vi "To CSV File.vi"(8 "error in (no error)":errorcluster, 9 "Path":path, 10 "engine configuration":refnum<class "engine configuration.lvclass">, 11 "DAQmx Module Editor Node in":refnum<class "DAQmx Module Editor Node.lvclass">) -> (0 "error out":errorcluster, 3 "DAQmx Module Editor Node out":refnum<class "DAQmx Module Editor Node.lvclass">)   [LabVIEW 2014, in "DAQmx Module Editor Node.lvclass"]
uses:
  DAQmx Module Editor Node.lvclass
  <vilib>/NI/Module Execution Interface/Engine Configuration/engine configuration.lvclass
  module/configuration/DAQmx Module Configuration.lvclass
  <vilib>/NI/Configuration Framework/serializable configuration/NISE_CEF_serializable configuration.lvclass/NISE_CEF_serializable configuration.ctl
  module/configuration/DAQmx Module Configuration.lvclass/DAQmx Module Configuration.ctl
  <vilib>/NI/Tag Bus/tag/tag descriptor.lvclass/tag descriptor.ctl
  <vilib>/Utility/LVClass/Get LV Class Name.vi
  <vilib>/NI/Configuration Framework/error generator/NISE_error generator.vi
  <vilib>/NI/Configuration Framework/serializable configuration/NISE_CEF_serializable configuration.lvclass
  <vilib>/NI/Tag Bus Module Framework/channel/TBM channel.lvclass
  <vilib>/NI/Tag Bus/tag/tag descriptor.lvclass
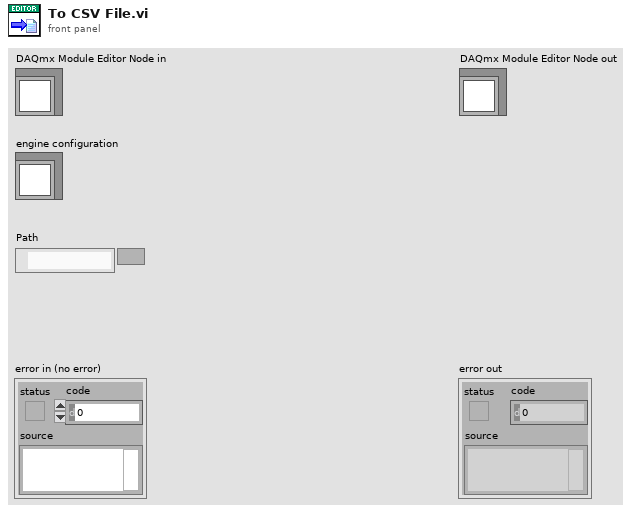
[diagram p1: front panel]
types:
  T1 = typedef "DAQmx Module Configuration.lvclass/Line.ctl" = cluster{"channel":refnum<class "TBM channel.lvclass">, "Physical Channel":string, "Measurement Type":T2, "Parameters":T3}
  T2 = typedef "DAQmx Module Configuration.lvclass/Measurement Type.ctl" = enum16{"Digital Input", "Digital Output", "Voltage Input", "Voltage Output", "Current Input", "Current Output", "RTD", "Thermocouple", "Strain"}
  T3 = typedef "DAQmx Module Configuration.lvclass/Parameters.ctl" = cluster{"Digital Config":cluster{"Invert Lines?":bool}, "Voltage Config":cluster{"Maximum Value (V)":dbl, "Minimum Value (V)":dbl, "in terminal configuration (V)":i32, "out terminal configuration (V)":i32}, "Current Config":cluster{"Maximum Value (A)":dbl, "Minimum Value (A)":dbl, "shunt resistor location":i32, "input terminal configuration (C)":i32, "external shunt resistor value":dbl}, "RTD Config":cluster{"Maximum Value (°C)":dbl, "Minimum Value (°C)":dbl, "resistance configuration":i32, "r0":dbl, "current excitation value":dbl, "rtd type":i32, "current excitation source":i32}, "Thermocouple Config":cluster{"Minimum Value (C)":dbl, "Maximum Value (C)":dbl, "thermocouple type":i32, "cjc source":i32, "cjc value":dbl}, "Strain Config":cluster{"Maximum Value":dbl, "Minimum Value":dbl, "bridge information":cluster{"strain configuration":i32, "lead wire resistance":dbl, "initial bridge voltage":dbl, "voltage excitation source":i32, "voltage excitation value":dbl}, "strain gage information":cluster{"gage factor":dbl, "nominal gage resistance":dbl, "poisson ratio":dbl}}}
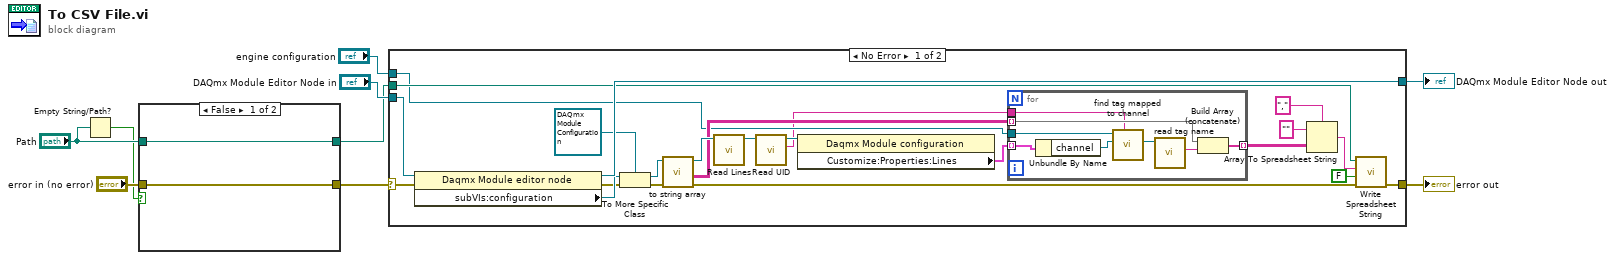
[diagram p0: block diagram]
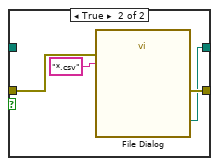
[diagram p2: hidden frame]
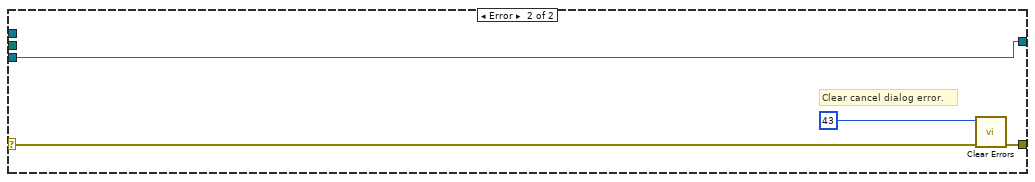
[diagram p3: hidden frame]
diagram:
  n1 = Empty String/Path?(string/path="Path") -> (empty?=w1:bool)
  n2 = case shown="False" w1 {
    tunnel: "error in (no error)" -> [w10 w14]
    tunnel: [w10 w13] -> w4
    tunnel: [w11 w12] -> w3
    tunnel: "Path" -> [w11 _]
    frame False {
    }
    frame True {
      n3 = call "File Dialog"("error in"=w14, "pattern (all files)"="*.csv") -> ("selected path"=w12:path, "error out"=w13:errorcluster)  [unwired: 10 in, 2 out]
    }
  }
  n4 = case shown="No Error" w4 {
    selector: w4 -> [w26 w49]
    tunnel: [w32 w48] -> w9
    tunnel: [w37 w50] -> w6
    tunnel: "DAQmx Module Editor Node in" -> [w38 w50]
    tunnel: w3 -> [w27 _]
    tunnel: "engine configuration" -> [w18 _]
    frame No Error {
      n5 = property class="Daqmx Module editor node"(reference=w38, error in=w26) -> (reference out=w37:refnum<class "DAQmx Module Editor Node.lvclass">, error out=w28:errorcluster, "subVIs:configuration"=w36:refnum<class "NISE_CEF_serializable configuration.lvclass">)
      n6 = To More Specific Class(target class=refnum<class "DAQmx Module Configuration.lvclass"> refnum ("Daqmx Module configuration out"), reference=w36, error in=w28) -> (specific class reference=w35:refnum<class "DAQmx Module Configuration.lvclass">, error out=w34:errorcluster)
      n7 = call-dynamic "to string array.vi"("error in (no error)"=w34, "module configuration in"=w35) -> ("error out"=w33:errorcluster, "Array"=w22:string[][], "module configuration out"=w25:refnum<class "DAQmx Module Configuration.lvclass">)  [unwired: 6 in, 1 out]
      n8 = call "Read Lines.vi"("Daqmx Module configuration in"=w25) -> ("Daqmx Module configuration out"=w23:refnum<class "DAQmx Module Configuration.lvclass">)  [unwired: 8 in, 2 out]
      n9 = call <vilib>:"Read UID.vi"("configuration in"=w23) -> ("instance id"=w17:string, "configuration out"=w20:refnum<class "DAQmx Module Configuration.lvclass">)  [unwired: 8 in, 1 out]
      n10 = property class="Daqmx Module configuration"(reference=w20) -> ("Customize:Properties:Lines"=w19:T1[])  [unwired: 1 in, 2 out]
      n11 = for {
        tunnel: w22 -> [w42] mode=indexing
        tunnel: [w40] -> w21 mode=indexing
        tunnel: w19 -> [w46] mode=indexing
        tunnel: w18 -> [w44]
        tunnel: w17 -> [w39]
        n12 = Unbundle By Name(w46) -> ("channel"=w45:refnum<class "TBM channel.lvclass">)
        n13 = call <vilib>:"find tag mapped to channel.vi"("owner"=w39, "channel"=w45, "engine configuration in"=w44) -> ("tag"=w43:refnum<class "tag descriptor.lvclass">)  [unwired: 6 in, 2 out]
        n14 = call <vilib>:"read tag name.vi"("system tag in"=w43) -> ("name"=w41:string)  [unwired: 8 in, 2 out]
        n15 = Build Array (concatenate)(w42, w41) -> (w40:string[])
      }
      n16 = Array To Spreadsheet String(delimiter (Tab)=",", array=w21, 3:"" ("format string")) -> (spreadsheet string=w31:string)
      n17 = call <vilib>:"Write Spreadsheet String.vi"("error in"=w33, "append to file? (new file:F)"=FALSE, "spreadsheet string"=w31, "file path (dialog if empty)"=w27) -> ("error out"=w32:errorcluster)  [unwired: 6 in, 1 out]
    }
    frame Error {
      # "Clear cancel dialog error."
      n18 = call <vilib>:"Clear Errors.vi"("error in (no error)"=w49, "specific error code to clear (0: all)"=43) -> ("error out"=w48:errorcluster)  [unwired: 4 in, 1 out]
    }
  }
  "error out" <- w9
  "DAQmx Module Editor Node out" <- w6
